vi "Program.vi"() -> ()   [LabVIEW 2026]
uses:
  <instrlib>/MicroPulse/Public/Data/Datatypes/MP - pulse damping.ctl
  <instrlib>/MicroPulse/Public/Data/Datatypes/MP - frequency filter.ctl
  <instrlib>/MicroPulse/Public/Data/Datatypes/MP - sample frequency.ctl
  <instrlib>/MicroPulse/Public/Data/Datatypes/TCP config.ctl
  <instrlib>/MicroPulse/Public/Data/Datatypes/MP - test parameters.ctl
  <instrlib>/MicroPulse/Public/Data/Datatypes/MP - transmit parameters.ctl
  <instrlib>/MicroPulse/Public/Data/Datatypes/MP - pulser voltage.ctl
  <instrlib>/MicroPulse/Public/Data/Datatypes/MP - receive parameters.ctl
  <instrlib>/MicroPulse/Public/Data/Datatypes/MP - display gate.ctl
  <instrlib>/MicroPulse/Public/Data/Datatypes/MP - waveform type.ctl
  <instrlib>/MicroPulse/Public/Data/Datatypes/MP - analogue filter.ctl
  <instrlib>/MicroPulse/Public/Data/Datatypes/MP - digital filtering.ctl
  <instrlib>/MicroPulse/Public/Data/Datatypes/MP - high pass filter.ctl
  <instrlib>/MicroPulse/Public/Data/Datatypes/MP - low pass filter.ctl
  <instrlib>/MicroPulse/Public/Data/Datatypes/MP - multi-gate inspection.ctl
  <instrlib>/MicroPulse/Public/Data/Datatypes/MP - multigate inspection gate parameters.ctl
  <instrlib>/MicroPulse/Public/Data/Datatypes/MP - hysteresis level.ctl
  <instrlib>/MicroPulse/Public/Data/Datatypes/MP - multigate mode.ctl
  <instrlib>/MicroPulse/Public/Data/Datatypes/MP - data formatting.ctl
  <instrlib>/MicroPulse/Public/Data/Datatypes/MP - amplitude reporting mode.ctl
  <instrlib>/MicroPulse/Public/Data/Datatypes/MP - averaging.ctl
  <vilib>/ErrorRing/Error Ring.xnode
  <instrlib>/MicroPulse/MicroPulse_Driver.lvlib
panel:
  in  "Main Tab Control":T1(tab)
  in  "Calculate Scan":bool
  in  "Scan Information":T2 {"Date" format="%<%x>T"}
  in  "Scan Settings":T3={"Selected Beam X"=0.0, "Enabled Channels"=1.0, "Scan Data Rate"=0.0, "Scan Resolution"=0.0, "Scan Speed (deg/s)"=0.0, "Scan RPM"=0.0, "Pulses Per Rev"=0.0} {"Enabled Channels" min=1.0 max=7.0 step=1.0 format="%#.0f"}
  in  "Transducer Information":string[][](table)
  in  "Gain Slider":dbl(slide) caption="Gain (dB)" min=0.0 max=50.0 step=0.25 scale=0.0..50.0
  in  "Channel Setup Tab Control":T4(tab)
  in  "Pulse Width Damping Channel 1":T7
  in  "Interface Channel 1":T8
  out "Flaw Indicators Channel 1":T9
  in  "Flaw Gate Channel 1":T8 caption="Flaw Gate (mm Ti)"
  in  "Backwall Gate Channel 1":T8 caption="Backwall Gate (mm)"
  in  "A-Scan Window Channel 1":cluster{"Start":dbl, "Range":dbl} caption="A-Scan Window (mm)"
  in  "Pulse Width Damping Channel 2":T7
  in  "Interface Channel 2":T8
  out "Flaw Indicators Channel 2":T9
  in  "Flaw Gate Channel 2":T8 caption="Flaw Gate (mm Ti)"
  in  "Backwall Gate Channel 2":T8 caption="Backwall Gate (mm)"
  in  "A-Scan Window Channel 2":cluster{"Start":dbl, "Range":dbl} caption="A-Scan Window (mm)"
  in  "Pulse Width Damping Channel 3":T7
  in  "Interface Channel 3":T8
  out "Flaw Indicators Channel 3":T9
  in  "Flaw Gate Channel 3":T8 caption="Flaw Gate (mm Ti)"
  in  "Backwall Gate Channel 3":T8 caption="Backwall Gate (mm)"
  in  "A-Scan Window Channel 3":cluster{"Start":dbl, "Range":dbl} caption="A-Scan Window (mm)"
  in  "A-Scan Window Channel 4":cluster{"Start":dbl, "Range":dbl} caption="A-Scan Window (mm)"
  in  "Backwall Gate Channel 4":T8 caption="Backwall Gate (mm)"
  in  "Flaw Gate Channel 4":T8 caption="Flaw Gate (mm Ti)"
  out "Flaw Indicators Channel 4":T9
  in  "Interface Channel 4":T8
  in  "Pulse Width Damping Channel 4":T7
  in  "Pulse Width Damping Channel 5":T7
  in  "Interface Channel 5":T8
  out "Flaw Indicators Channel 5":T9
  in  "Flaw Gate Channel 5":T8 caption="Flaw Gate (mm Ti)"
  in  "Backwall Gate Channel 5":T8 caption="Backwall Gate (mm)"
  in  "A-Scan Window Channel 5":cluster{"Start":dbl, "Range":dbl} caption="A-Scan Window (mm)"
  in  "Pulse Width Damping Channel 6":T7
  in  "Interface Channel 6":T8
  out "Flaw Indicators Channel 6":T9
  in  "Flaw Gate Channel 6":T8 caption="Flaw Gate (mm Ti)"
  in  "Backwall Gate Channel 6":T8 caption="Backwall Gate (mm)"
  in  "A-Scan Window Channel 6":cluster{"Start":dbl, "Range":dbl} caption="A-Scan Window (mm)"
  in  "Pulse Width Damping Channel 7":T7
  in  "Interface Channel 7":T8
  out "Flaw Indicators Channel 7":T9
  in  "Flaw Gate Channel 7":T8 caption="Flaw Gate (mm Ti)"
  in  "Backwall Gate Channel 7":T8 caption="Backwall Gate (mm)"
  in  "A-Scan Window Channel 7":cluster{"Start":dbl, "Range":dbl} caption="A-Scan Window (mm)"
  out "Channel Setup Graph":cluster{"timebase":dbl[], "data":u16[]}[](graph)
  in  "Channel Select":T10(ring)
  in  "Channel Variables Tab Control":T4(tab)
  in  "RX Channel 1":T11 {"Delay" format="%#_g us"; "Display Gate"."Length" min=0.0 max=64000.0 step=1.0 format="%#_g us"; "Display Gate"."Start" min=0.0 max=64000.0 step=1.0 format="%#_g us"; "Analogue Filtering"."Smoothing" min=1 max=11 step=1; "Gain" min=-6.0 max=70.0 step=0.25 format="%.2fdB"}
  in  "Test Channel 1":T18={"Test No."=1, "Tx Channel"=1, "Rx Channel"=1} {"Rx Channel" min=1 max=1024; "Tx Channel" min=1 max=1024}
  in  "TX Channel 1":T19 {"Pulse Shape"."Width" min=16 max=1010 step=50 format="%.0fns"}
  in  "Data Format Channel 1":T21={"Amplitude Mode"=enum."Peaks + Ascan for Multigate", "Averaging"=enum."None", "Coupling Level"=0} {"Coupling Level" max=4095 step=1}
  in  "Gates Channel 1":T24={"Gate 1"={"Start (us)"=0.0, "Length (us)"=0.0, "Threshold"=10, "Enabled?"=FALSE, "Max # Peaks"=0, "Hysteresis"=enum."None", "Mode"=enum."1st Peak in Gate", "Inverted?"=FALSE, "Colour "=0}, "Gate 2"={"Start (us)"=0.0, "Length (us)"=0.0, "Threshold"=10, "Enabled?"=FALSE, "Max # Peaks"=0, "Hysteresis"=enum."None", "Mode"=enum."1st Peak in Gate", "Inverted?"=FALSE, "Colour "=0}, "Gate 3"={"Start (us)"=0.0, "Length (us)"=0.0, "Threshold"=10, "Enabled?"=FALSE, "Max # Peaks"=0, "Hysteresis"=enum."None", "Mode"=enum."1st Peak in Gate", "Inverted?"=FALSE, "Colour "=0}, "Gate 4"={"Start (us)"=0.0, "Length (us)"=0.0, "Threshold"=10, "Enabled?"=FALSE, "Max # Peaks"=0, "Hysteresis"=enum."None", "Mode"=enum."1st Peak in Gate", "Inverted?"=FALSE, "Colour "=0}} {"Gate 4"."Max # Peaks" max=64000 step=100; "Gate 4"."Threshold" min=10 max=4095 step=10; "Gate 4"."Length (us)" min=0.0 max=96000.0 step=100.0; "Gate 4"."Start (us)" min=0.0 max=64000.0 step=100.0; "Gate 3"."Max # Peaks" max=64000 step=100; "Gate 3"."Threshold" min=10 max=4095 step=10; "Gate 3"."Length (us)" min=0.0 max=96000.0 step=100.0; "Gate 3"."Start (us)" min=0.0 max=64000.0 step=100.0; "Gate 2"."Max # Peaks" max=64000 step=100; "Gate 2"."Threshold" min=10 max=4095 step=10; "Gate 2"."Length (us)" min=0.0 max=96000.0 step=100.0; "Gate 2"."Start (us)" min=0.0 max=64000.0 step=100.0; "Gate 1"."Max # Peaks" max=64000 step=100; "Gate 1"."Threshold" min=10 max=4095 step=10; "Gate 1"."Length (us)" min=0.0 max=96000.0 step=100.0; "Gate 1"."Start (us)" min=0.0 max=64000.0 step=100.0}
  in  "Gates Channel 2":T24={"Gate 1"={"Start (us)"=0.0, "Length (us)"=0.0, "Threshold"=10, "Enabled?"=FALSE, "Max # Peaks"=0, "Hysteresis"=enum."None", "Mode"=enum."1st Peak in Gate", "Inverted?"=FALSE, "Colour "=0}, "Gate 2"={"Start (us)"=0.0, "Length (us)"=0.0, "Threshold"=10, "Enabled?"=FALSE, "Max # Peaks"=0, "Hysteresis"=enum."None", "Mode"=enum."1st Peak in Gate", "Inverted?"=FALSE, "Colour "=0}, "Gate 3"={"Start (us)"=0.0, "Length (us)"=0.0, "Threshold"=10, "Enabled?"=FALSE, "Max # Peaks"=0, "Hysteresis"=enum."None", "Mode"=enum."1st Peak in Gate", "Inverted?"=FALSE, "Colour "=0}, "Gate 4"={"Start (us)"=0.0, "Length (us)"=0.0, "Threshold"=10, "Enabled?"=FALSE, "Max # Peaks"=0, "Hysteresis"=enum."None", "Mode"=enum."1st Peak in Gate", "Inverted?"=FALSE, "Colour "=0}} {"Gate 4"."Max # Peaks" max=64000 step=100; "Gate 4"."Threshold" min=10 max=4095 step=10; "Gate 4"."Length (us)" min=0.0 max=96000.0 step=100.0; "Gate 4"."Start (us)" min=0.0 max=64000.0 step=100.0; "Gate 3"."Max # Peaks" max=64000 step=100; "Gate 3"."Threshold" min=10 max=4095 step=10; "Gate 3"."Length (us)" min=0.0 max=96000.0 step=100.0; "Gate 3"."Start (us)" min=0.0 max=64000.0 step=100.0; "Gate 2"."Max # Peaks" max=64000 step=100; "Gate 2"."Threshold" min=10 max=4095 step=10; "Gate 2"."Length (us)" min=0.0 max=96000.0 step=100.0; "Gate 2"."Start (us)" min=0.0 max=64000.0 step=100.0; "Gate 1"."Max # Peaks" max=64000 step=100; "Gate 1"."Threshold" min=10 max=4095 step=10; "Gate 1"."Length (us)" min=0.0 max=96000.0 step=100.0; "Gate 1"."Start (us)" min=0.0 max=64000.0 step=100.0}
  in  "Data Format Channel 2":T21={"Amplitude Mode"=enum."Peaks + Ascan for Multigate", "Averaging"=enum."None", "Coupling Level"=0} {"Coupling Level" max=4095 step=1}
  in  "TX Channel 2":T19 {"Pulse Shape"."Width" min=16 max=1010 step=50 format="%.0fns"}
  in  "Test Channel 2":T18={"Test No."=2, "Tx Channel"=2, "Rx Channel"=2} {"Rx Channel" min=1 max=1024; "Tx Channel" min=1 max=1024}
  in  "RX Channel 2":T11 {"Delay" format="%#_g us"; "Display Gate"."Length" min=0.0 max=64000.0 step=1.0 format="%#_g us"; "Display Gate"."Start" min=0.0 max=64000.0 step=1.0 format="%#_g us"; "Analogue Filtering"."Smoothing" min=1 max=11 step=1; "Gain" min=-6.0 max=70.0 step=0.25 format="%.2fdB"}
  in  "Gates Channel 3":T24={"Gate 1"={"Start (us)"=0.0, "Length (us)"=0.0, "Threshold"=10, "Enabled?"=FALSE, "Max # Peaks"=0, "Hysteresis"=enum."None", "Mode"=enum."1st Peak in Gate", "Inverted?"=FALSE, "Colour "=0}, "Gate 2"={"Start (us)"=0.0, "Length (us)"=0.0, "Threshold"=10, "Enabled?"=FALSE, "Max # Peaks"=0, "Hysteresis"=enum."None", "Mode"=enum."1st Peak in Gate", "Inverted?"=FALSE, "Colour "=0}, "Gate 3"={"Start (us)"=0.0, "Length (us)"=0.0, "Threshold"=10, "Enabled?"=FALSE, "Max # Peaks"=0, "Hysteresis"=enum."None", "Mode"=enum."1st Peak in Gate", "Inverted?"=FALSE, "Colour "=0}, "Gate 4"={"Start (us)"=0.0, "Length (us)"=0.0, "Threshold"=10, "Enabled?"=FALSE, "Max # Peaks"=0, "Hysteresis"=enum."None", "Mode"=enum."1st Peak in Gate", "Inverted?"=FALSE, "Colour "=0}} {"Gate 4"."Max # Peaks" max=64000 step=100; "Gate 4"."Threshold" min=10 max=4095 step=10; "Gate 4"."Length (us)" min=0.0 max=96000.0 step=100.0; "Gate 4"."Start (us)" min=0.0 max=64000.0 step=100.0; "Gate 3"."Max # Peaks" max=64000 step=100; "Gate 3"."Threshold" min=10 max=4095 step=10; "Gate 3"."Length (us)" min=0.0 max=96000.0 step=100.0; "Gate 3"."Start (us)" min=0.0 max=64000.0 step=100.0; "Gate 2"."Max # Peaks" max=64000 step=100; "Gate 2"."Threshold" min=10 max=4095 step=10; "Gate 2"."Length (us)" min=0.0 max=96000.0 step=100.0; "Gate 2"."Start (us)" min=0.0 max=64000.0 step=100.0; "Gate 1"."Max # Peaks" max=64000 step=100; "Gate 1"."Threshold" min=10 max=4095 step=10; "Gate 1"."Length (us)" min=0.0 max=96000.0 step=100.0; "Gate 1"."Start (us)" min=0.0 max=64000.0 step=100.0}
  in  "Data Format Channel 3":T21={"Amplitude Mode"=enum."Peaks + Ascan for Multigate", "Averaging"=enum."None", "Coupling Level"=0} {"Coupling Level" max=4095 step=1}
  in  "TX Channel 3":T19 {"Pulse Shape"."Width" min=16 max=1010 step=50 format="%.0fns"}
  in  "Test Channel 3":T18={"Test No."=3, "Tx Channel"=3, "Rx Channel"=3} {"Rx Channel" min=1 max=1024; "Tx Channel" min=1 max=1024}
  in  "RX Channel 3":T11 {"Delay" format="%#_g us"; "Display Gate"."Length" min=0.0 max=64000.0 step=1.0 format="%#_g us"; "Display Gate"."Start" min=0.0 max=64000.0 step=1.0 format="%#_g us"; "Analogue Filtering"."Smoothing" min=1 max=11 step=1; "Gain" min=-6.0 max=70.0 step=0.25 format="%.2fdB"}
  in  "RX Channel 4":T11 {"Delay" format="%#_g us"; "Display Gate"."Length" min=0.0 max=64000.0 step=1.0 format="%#_g us"; "Display Gate"."Start" min=0.0 max=64000.0 step=1.0 format="%#_g us"; "Analogue Filtering"."Smoothing" min=1 max=11 step=1; "Gain" min=-6.0 max=70.0 step=0.25 format="%.2fdB"}
  in  "Test Channel 4":T18={"Test No."=4, "Tx Channel"=4, "Rx Channel"=4} {"Rx Channel" min=1 max=1024; "Tx Channel" min=1 max=1024}
  in  "TX Channel 4":T19 {"Pulse Shape"."Width" min=16 max=1010 step=50 format="%.0fns"}
  in  "Data Format Channel 4":T21={"Amplitude Mode"=enum."Peaks + Ascan for Multigate", "Averaging"=enum."None", "Coupling Level"=0} {"Coupling Level" max=4095 step=1}
  in  "Gates Channel 4":T24={"Gate 1"={"Start (us)"=0.0, "Length (us)"=0.0, "Threshold"=10, "Enabled?"=FALSE, "Max # Peaks"=0, "Hysteresis"=enum."None", "Mode"=enum."1st Peak in Gate", "Inverted?"=FALSE, "Colour "=0}, "Gate 2"={"Start (us)"=0.0, "Length (us)"=0.0, "Threshold"=10, "Enabled?"=FALSE, "Max # Peaks"=0, "Hysteresis"=enum."None", "Mode"=enum."1st Peak in Gate", "Inverted?"=FALSE, "Colour "=0}, "Gate 3"={"Start (us)"=0.0, "Length (us)"=0.0, "Threshold"=10, "Enabled?"=FALSE, "Max # Peaks"=0, "Hysteresis"=enum."None", "Mode"=enum."1st Peak in Gate", "Inverted?"=FALSE, "Colour "=0}, "Gate 4"={"Start (us)"=0.0, "Length (us)"=0.0, "Threshold"=10, "Enabled?"=FALSE, "Max # Peaks"=0, "Hysteresis"=enum."None", "Mode"=enum."1st Peak in Gate", "Inverted?"=FALSE, "Colour "=0}} {"Gate 4"."Max # Peaks" max=64000 step=100; "Gate 4"."Threshold" min=10 max=4095 step=10; "Gate 4"."Length (us)" min=0.0 max=96000.0 step=100.0; "Gate 4"."Start (us)" min=0.0 max=64000.0 step=100.0; "Gate 3"."Max # Peaks" max=64000 step=100; "Gate 3"."Threshold" min=10 max=4095 step=10; "Gate 3"."Length (us)" min=0.0 max=96000.0 step=100.0; "Gate 3"."Start (us)" min=0.0 max=64000.0 step=100.0; "Gate 2"."Max # Peaks" max=64000 step=100; "Gate 2"."Threshold" min=10 max=4095 step=10; "Gate 2"."Length (us)" min=0.0 max=96000.0 step=100.0; "Gate 2"."Start (us)" min=0.0 max=64000.0 step=100.0; "Gate 1"."Max # Peaks" max=64000 step=100; "Gate 1"."Threshold" min=10 max=4095 step=10; "Gate 1"."Length (us)" min=0.0 max=96000.0 step=100.0; "Gate 1"."Start (us)" min=0.0 max=64000.0 step=100.0}
  in  "RX Channel 5":T11 {"Delay" format="%#_g us"; "Display Gate"."Length" min=0.0 max=64000.0 step=1.0 format="%#_g us"; "Display Gate"."Start" min=0.0 max=64000.0 step=1.0 format="%#_g us"; "Analogue Filtering"."Smoothing" min=1 max=11 step=1; "Gain" min=-6.0 max=70.0 step=0.25 format="%.2fdB"}
  in  "Test Channel 5":T18={"Test No."=5, "Tx Channel"=5, "Rx Channel"=5} {"Rx Channel" min=1 max=1024; "Tx Channel" min=1 max=1024}
  in  "TX Channel 5":T19 {"Pulse Shape"."Width" min=16 max=1010 step=50 format="%.0fns"}
  in  "Data Format Channel 5":T21={"Amplitude Mode"=enum."Peaks + Ascan for Multigate", "Averaging"=enum."None", "Coupling Level"=0} {"Coupling Level" max=4095 step=1}
  in  "Gates Channel 5":T24={"Gate 1"={"Start (us)"=0.0, "Length (us)"=0.0, "Threshold"=10, "Enabled?"=FALSE, "Max # Peaks"=0, "Hysteresis"=enum."None", "Mode"=enum."1st Peak in Gate", "Inverted?"=FALSE, "Colour "=0}, "Gate 2"={"Start (us)"=0.0, "Length (us)"=0.0, "Threshold"=10, "Enabled?"=FALSE, "Max # Peaks"=0, "Hysteresis"=enum."None", "Mode"=enum."1st Peak in Gate", "Inverted?"=FALSE, "Colour "=0}, "Gate 3"={"Start (us)"=0.0, "Length (us)"=0.0, "Threshold"=10, "Enabled?"=FALSE, "Max # Peaks"=0, "Hysteresis"=enum."None", "Mode"=enum."1st Peak in Gate", "Inverted?"=FALSE, "Colour "=0}, "Gate 4"={"Start (us)"=0.0, "Length (us)"=0.0, "Threshold"=10, "Enabled?"=FALSE, "Max # Peaks"=0, "Hysteresis"=enum."None", "Mode"=enum."1st Peak in Gate", "Inverted?"=FALSE, "Colour "=0}} {"Gate 4"."Max # Peaks" max=64000 step=100; "Gate 4"."Threshold" min=10 max=4095 step=10; "Gate 4"."Length (us)" min=0.0 max=96000.0 step=100.0; "Gate 4"."Start (us)" min=0.0 max=64000.0 step=100.0; "Gate 3"."Max # Peaks" max=64000 step=100; "Gate 3"."Threshold" min=10 max=4095 step=10; "Gate 3"."Length (us)" min=0.0 max=96000.0 step=100.0; "Gate 3"."Start (us)" min=0.0 max=64000.0 step=100.0; "Gate 2"."Max # Peaks" max=64000 step=100; "Gate 2"."Threshold" min=10 max=4095 step=10; "Gate 2"."Length (us)" min=0.0 max=96000.0 step=100.0; "Gate 2"."Start (us)" min=0.0 max=64000.0 step=100.0; "Gate 1"."Max # Peaks" max=64000 step=100; "Gate 1"."Threshold" min=10 max=4095 step=10; "Gate 1"."Length (us)" min=0.0 max=96000.0 step=100.0; "Gate 1"."Start (us)" min=0.0 max=64000.0 step=100.0}
  in  "RX Channel 6":T11 {"Delay" format="%#_g us"; "Display Gate"."Length" min=0.0 max=64000.0 step=1.0 format="%#_g us"; "Display Gate"."Start" min=0.0 max=64000.0 step=1.0 format="%#_g us"; "Analogue Filtering"."Smoothing" min=1 max=11 step=1; "Gain" min=-6.0 max=70.0 step=0.25 format="%.2fdB"}
  in  "Test Channel 6":T18={"Test No."=6, "Tx Channel"=6, "Rx Channel"=6} {"Rx Channel" min=1 max=1024; "Tx Channel" min=1 max=1024}
  in  "TX Channel 6":T19 {"Pulse Shape"."Width" min=16 max=1010 step=50 format="%.0fns"}
  in  "Data Format Channel 6":T21={"Amplitude Mode"=enum."Peaks + Ascan for Multigate", "Averaging"=enum."None", "Coupling Level"=0} {"Coupling Level" max=4095 step=1}
  in  "Gates Channel 6":T24={"Gate 1"={"Start (us)"=0.0, "Length (us)"=0.0, "Threshold"=10, "Enabled?"=FALSE, "Max # Peaks"=0, "Hysteresis"=enum."None", "Mode"=enum."1st Peak in Gate", "Inverted?"=FALSE, "Colour "=0}, "Gate 2"={"Start (us)"=0.0, "Length (us)"=0.0, "Threshold"=10, "Enabled?"=FALSE, "Max # Peaks"=0, "Hysteresis"=enum."None", "Mode"=enum."1st Peak in Gate", "Inverted?"=FALSE, "Colour "=0}, "Gate 3"={"Start (us)"=0.0, "Length (us)"=0.0, "Threshold"=10, "Enabled?"=FALSE, "Max # Peaks"=0, "Hysteresis"=enum."None", "Mode"=enum."1st Peak in Gate", "Inverted?"=FALSE, "Colour "=0}, "Gate 4"={"Start (us)"=0.0, "Length (us)"=0.0, "Threshold"=10, "Enabled?"=FALSE, "Max # Peaks"=0, "Hysteresis"=enum."None", "Mode"=enum."1st Peak in Gate", "Inverted?"=FALSE, "Colour "=0}} {"Gate 4"."Max # Peaks" max=64000 step=100; "Gate 4"."Threshold" min=10 max=4095 step=10; "Gate 4"."Length (us)" min=0.0 max=96000.0 step=100.0; "Gate 4"."Start (us)" min=0.0 max=64000.0 step=100.0; "Gate 3"."Max # Peaks" max=64000 step=100; "Gate 3"."Threshold" min=10 max=4095 step=10; "Gate 3"."Length (us)" min=0.0 max=96000.0 step=100.0; "Gate 3"."Start (us)" min=0.0 max=64000.0 step=100.0; "Gate 2"."Max # Peaks" max=64000 step=100; "Gate 2"."Threshold" min=10 max=4095 step=10; "Gate 2"."Length (us)" min=0.0 max=96000.0 step=100.0; "Gate 2"."Start (us)" min=0.0 max=64000.0 step=100.0; "Gate 1"."Max # Peaks" max=64000 step=100; "Gate 1"."Threshold" min=10 max=4095 step=10; "Gate 1"."Length (us)" min=0.0 max=96000.0 step=100.0; "Gate 1"."Start (us)" min=0.0 max=64000.0 step=100.0}
  in  "RX Channel 7":T11 {"Delay" format="%#_g us"; "Display Gate"."Length" min=0.0 max=64000.0 step=1.0 format="%#_g us"; "Display Gate"."Start" min=0.0 max=64000.0 step=1.0 format="%#_g us"; "Analogue Filtering"."Smoothing" min=1 max=11 step=1; "Gain" min=-6.0 max=70.0 step=0.25 format="%.2fdB"}
  in  "Test Channel 7":T18={"Test No."=7, "Tx Channel"=7, "Rx Channel"=7} {"Rx Channel" min=1 max=1024; "Tx Channel" min=1 max=1024}
  in  "TX Channel 7":T19 {"Pulse Shape"."Width" min=16 max=1010 step=50 format="%.0fns"}
  in  "Data Format Channel 7":T21={"Amplitude Mode"=enum."Peaks + Ascan for Multigate", "Averaging"=enum."None", "Coupling Level"=0} {"Coupling Level" max=4095 step=1}
  in  "Gates Channel 7":T24={"Gate 1"={"Start (us)"=0.0, "Length (us)"=0.0, "Threshold"=10, "Enabled?"=FALSE, "Max # Peaks"=0, "Hysteresis"=enum."None", "Mode"=enum."1st Peak in Gate", "Inverted?"=FALSE, "Colour "=0}, "Gate 2"={"Start (us)"=0.0, "Length (us)"=0.0, "Threshold"=10, "Enabled?"=FALSE, "Max # Peaks"=0, "Hysteresis"=enum."None", "Mode"=enum."1st Peak in Gate", "Inverted?"=FALSE, "Colour "=0}, "Gate 3"={"Start (us)"=0.0, "Length (us)"=0.0, "Threshold"=10, "Enabled?"=FALSE, "Max # Peaks"=0, "Hysteresis"=enum."None", "Mode"=enum."1st Peak in Gate", "Inverted?"=FALSE, "Colour "=0}, "Gate 4"={"Start (us)"=0.0, "Length (us)"=0.0, "Threshold"=10, "Enabled?"=FALSE, "Max # Peaks"=0, "Hysteresis"=enum."None", "Mode"=enum."1st Peak in Gate", "Inverted?"=FALSE, "Colour "=0}} {"Gate 4"."Max # Peaks" max=64000 step=100; "Gate 4"."Threshold" min=10 max=4095 step=10; "Gate 4"."Length (us)" min=0.0 max=96000.0 step=100.0; "Gate 4"."Start (us)" min=0.0 max=64000.0 step=100.0; "Gate 3"."Max # Peaks" max=64000 step=100; "Gate 3"."Threshold" min=10 max=4095 step=10; "Gate 3"."Length (us)" min=0.0 max=96000.0 step=100.0; "Gate 3"."Start (us)" min=0.0 max=64000.0 step=100.0; "Gate 2"."Max # Peaks" max=64000 step=100; "Gate 2"."Threshold" min=10 max=4095 step=10; "Gate 2"."Length (us)" min=0.0 max=96000.0 step=100.0; "Gate 2"."Start (us)" min=0.0 max=64000.0 step=100.0; "Gate 1"."Max # Peaks" max=64000 step=100; "Gate 1"."Threshold" min=10 max=4095 step=10; "Gate 1"."Length (us)" min=0.0 max=96000.0 step=100.0; "Gate 1"."Start (us)" min=0.0 max=64000.0 step=100.0}
  in  "MicroPulse Initialise":T30={"Hard Reset?"=FALSE, "Sample Frequency"=enum."Use Default", "TCP config"={"Connection ID"=refnum, "IP address"="10.1.1.2", "host port"=1067, "OC timeout"=-1, "Read timeout"=0, "Write timeout"=0}, "PRF (Hz)"=0.0} {"TCP config"."Write timeout" format="%dms"; "TCP config"."Read timeout" format="%dms"; "TCP config"."OC timeout" format="%dms"}
  out "Key Held":bool
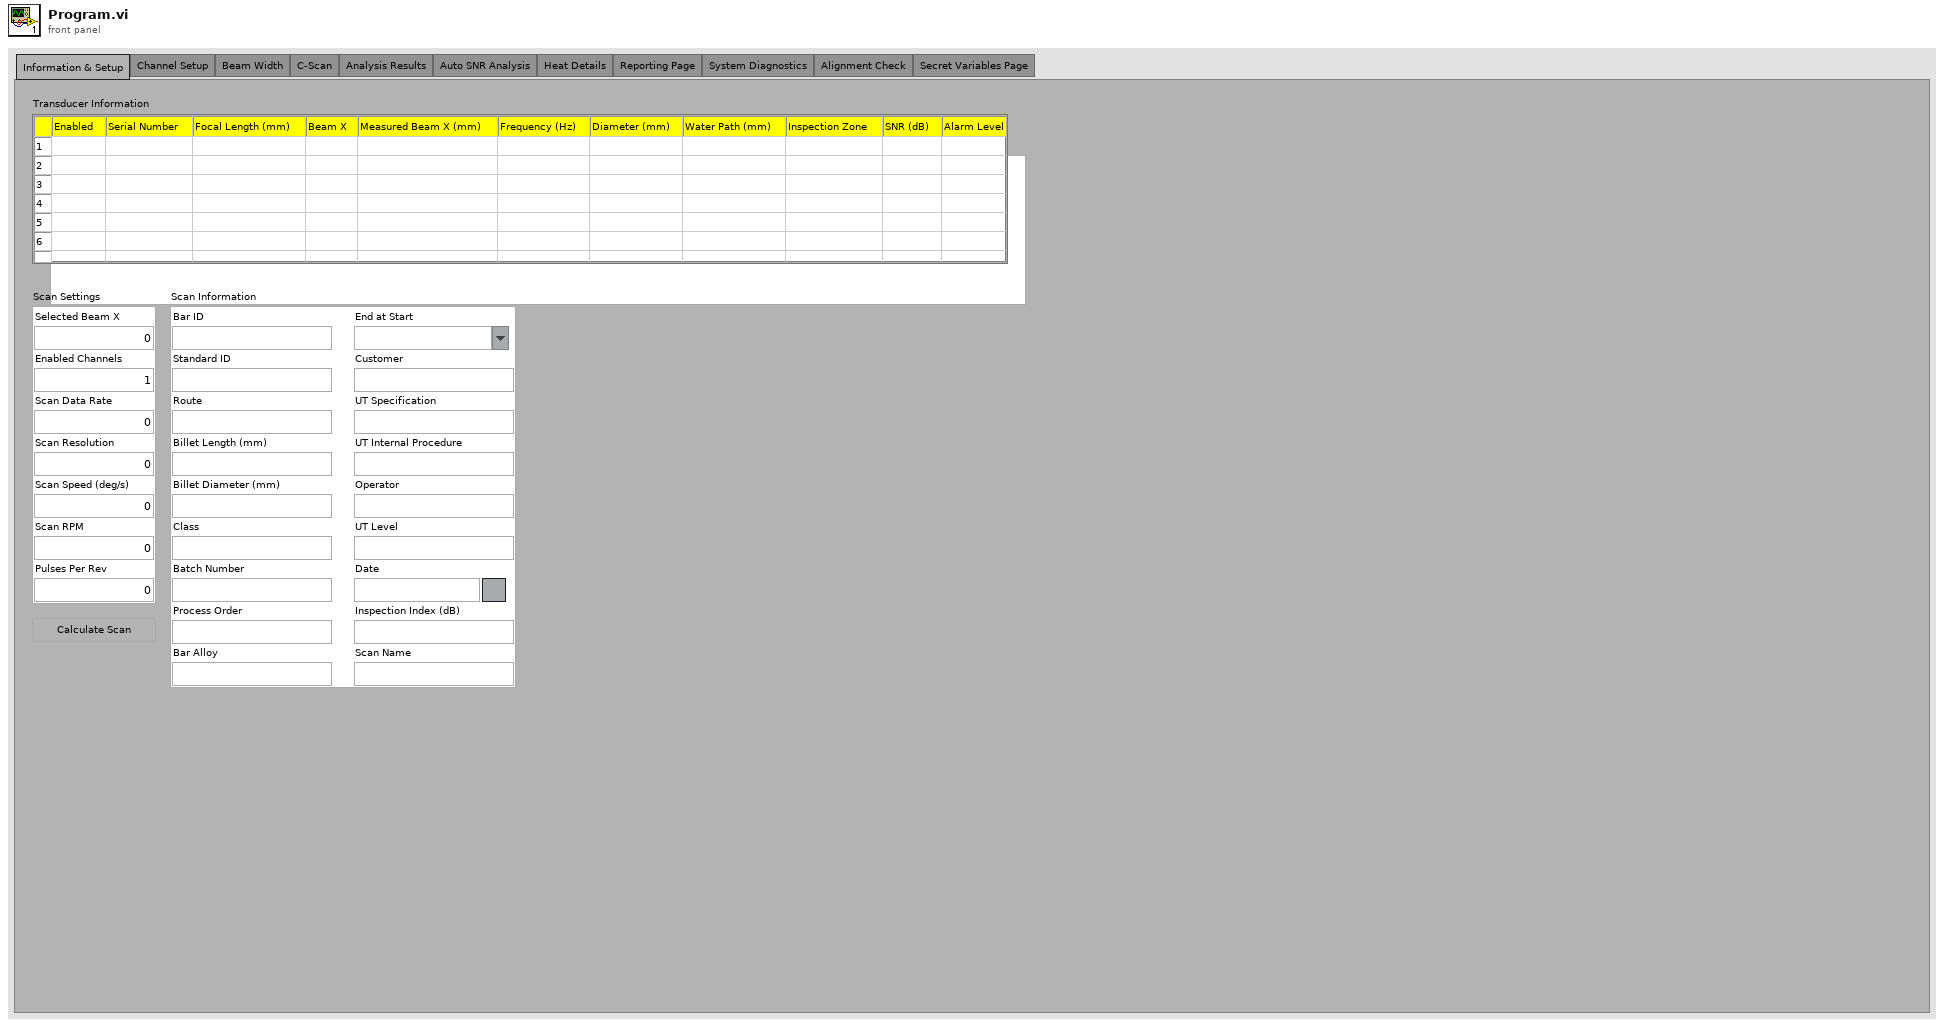
[diagram p1: front panel]
types:
  T1 = enum32{"Information & Setup", "Channel Setup", "Beam Width", "C-Scan", "Analysis Results", "Auto SNR Analysis", "Heat Details", "Reporting Page", "System Diagnostics", "Alignment Check", "Secret Variables Page"}
  T2 = cluster{"Bar ID":string, "Standard ID":string, "Route":string, "Billet Length (mm)":dbl, "Billet Diameter (mm)":dbl, "Class":string, "Batch Number":string, "Process Order":string, "Bar Alloy":string, "Scan Name":string, "Inspection Index (dB)":enum16{""}, "Date":timestamp, "UT Level":string, "Operator":string, "UT Internal Procedure":string, "UT Specification":string, "Customer":string, "End at Start":string}
  T3 = cluster{"Selected Beam X":dbl, "Enabled Channels":dbl, "Scan Data Rate":dbl, "Scan Resolution":dbl, "Scan Speed (deg/s)":dbl, "Scan RPM":dbl, "Pulses Per Rev":dbl}
  T4 = enum32{"Channel 1", "Channel 2", "Channel 3", "Channel 4", "Channel 5", "Channel 6", "Channel 7"}
  T5 = typedef "MicroPulse_Driver.lvlib/MP - pulse damping.ctl" = enum16{"660W", "458W", "220W", "149W", "102W", "82W", "63W", "51W"}
  T6 = typedef "MicroPulse_Driver.lvlib/MP - frequency filter.ctl" = enum16{"No change", "1MHz Bandpass", "2MHz Bandpass", "4MHz Bandpass", "5MHz Bandpass", "10MHz Bandpass", "2.5-18MHz Broadband", "0.75-12MHz  Broadband", "0.5MHz Bandpass", "5MHz 2nd Order TOFD", "10MHz 2nd Order TOFD", "3.0-25MHz Broadband", "3.0-30MHz Broadband"}
  T7 = cluster{"Pulse Width":dbl, "Damping Channel 1":T5, "Rectification":enum16{"Rectified Signal", "RF Signal", "+Half Wave", "-Half Wave"}, "Filter":T6}
  T8 = cluster{"Start":dbl, "Length":dbl, "Threshold":dbl}
  T9 = cluster{"Water Path":dbl, "Gate AMP":dbl, "Gate TOF":dbl}
  T10 = enum16{"Channel 1", "Channel 2", "Channel 3", "Channel 4", "Channel 5", "Channel 6", "Channel 7"}
  T11 = typedef "MicroPulse_Driver.lvlib/MP - receive parameters.ctl" = cluster{"Display Gate":T12, "Delay":dbl, "Waveform Type":T13, "Gain":dbl, "Analogue Filtering":T14, "Digital Filtering":T15}
  T12 = typedef "MicroPulse_Driver.lvlib/MP - display gate.ctl" = cluster{"Start":dbl, "Length":dbl}
  T13 = typedef "MicroPulse_Driver.lvlib/MP - waveform type.ctl" = enum16{"Rectified Signal", "RF Signal", "+Half Wave", "-Half Wave"}
  T14 = typedef "MicroPulse_Driver.lvlib/MP - analogue filter.ctl" = cluster{"Bandpass":T6, "Smoothing":u16}
  T15 = typedef "MicroPulse_Driver.lvlib/MP - digital filtering.ctl" = cluster{"High Pass Filter":T16, "Low Pass Filter":T17}
  T16 = typedef "MicroPulse_Driver.lvlib/MP - high pass filter.ctl" = enum16{"None", "0.7MHz", "1.5MHz", "4.0MHz", "7.5MHz", "10.0MHz", "User Defined"}
  T17 = typedef "MicroPulse_Driver.lvlib/MP - low pass filter.ctl" = enum16{"None", "1.8MHz", "3.0MHz", "6.0MHz", "8.0MHz", "12.0MHz", "User Defined"}
  T18 = typedef "MicroPulse_Driver.lvlib/MP - test parameters.ctl" = cluster{"Test No.":u32, "Tx Channel":u32, "Rx Channel":u32}
  T19 = typedef "MicroPulse_Driver.lvlib/MP - transmit parameters.ctl" = cluster{"Pulse Voltage":T20, "Pulse Shape":cluster{"Damping":T5, "Width":u32}}
  T20 = typedef "MicroPulse_Driver.lvlib/MP - pulser voltage.ctl" = enum16{"50V", "100V", "150V", "200V", "250V", "300V"}
  T21 = typedef "MicroPulse_Driver.lvlib/MP - data formatting.ctl" = cluster{"Amplitude Mode":T22, "Averaging":T23, "Coupling Level":u32}
  T22 = typedef "MicroPulse_Driver.lvlib/MP - amplitude reporting mode.ctl" = enum16{"1st Peak in gate", "Maximum Peak in gate", "All Peaks", "Ascan Data", "1st Threshold Crossing Peak", "Ascan + Peaks", "All Peaks for Multigate", "Peaks + Ascan for Multigate", "Peaks + P_Ascan for Multigate", "Full Matrix Capture"}
  T23 = typedef "MicroPulse_Driver.lvlib/MP - averaging.ctl" = enum16{"None", "2", "4", "8", "16", "32", "64", "128", "256"}
  T24 = typedef "MicroPulse_Driver.lvlib/MP - multi-gate inspection.ctl" = cluster{"Gate 1":T25, "Gate 2":T25, "Gate 3":T25, "Gate 4":T25}
  T25 = typedef "MicroPulse_Driver.lvlib/MP - multigate inspection gate parameters.ctl" = cluster{"Start (us)":dbl, "Length (us)":dbl, "Threshold":u16, "Enabled?":bool, "Max # Peaks":u16, "Hysteresis":T26, "Mode":T27, "Inverted?":bool, "Colour ":u32}
  T26 = typedef "MicroPulse_Driver.lvlib/MP - hysteresis level.ctl" = enum16{"None", "3dB", "6dB", "9dB", "12dB"}
  T27 = typedef "MicroPulse_Driver.lvlib/MP - multigate mode.ctl" = enum16{"1st Peak in Gate", "Largest Peak In Gate", "All Peaks In Gate", "1st Threshold Crossing"}
  T28 = typedef "MicroPulse_Driver.lvlib/MP - sample frequency.ctl" = enum16{"Use Default", "200MHz (LT2 only)", "100MHz", "50MHz", "25MHz", "10MHz"}
  T29 = typedef "MicroPulse_Driver.lvlib/TCP config.ctl" = cluster{"Connection ID":refnum<k5>, "IP address":string, "host port":u16, "OC timeout":i32, "Read timeout":i32, "Write timeout":i32}
  T30 = cluster{"Hard Reset?":bool, "Sample Frequency":T28, "TCP config":T29, "PRF (Hz)":dbl}
  T31 = enum16{"Init Program", "Init Hardware", "Main", "Reset", "Shutdown"}
  T32 = typedef "MicroPulse_Driver.lvlib/MP - scan data info.ctl" = cluster{"Message Header":u16, "Error Message":u16, "Test No.":u32, "Channel No.":u8, "Sweep No.":u32, "Gate No.":u32, "DOF":T33, "retain data":T34, "scan data":u16[], "scan length":i32, "scan index":i32, "peak data":cluster{"timebase":u16[], "data":u16[]}, "#peaks":i32, "PRF":dbl, "IP":cluster{"Axis No.":u8, "Location":u32, "MIP location":u32, "MIP?":bool}, "echo range":u16, "ETG":bool, "CAL 0 complete":bool, "Axis Positions":T35}
  T33 = typedef "MicroPulse_Driver.lvlib/MP - data output format.ctl" = enum16{"", "8-bit Mode", "10-bit Mode", "12-bit Mode", "16-bit Mode", "8-bit Log Mode", "12-bit Packed Mode"}
  T34 = typedef "MicroPulse_Driver.lvlib/MP - retain scan.ctl" = enum16{"None", "Ascan", "Peaks"}
  T35 = typedef "MicroPulse_Driver.lvlib/MP - axis positions (LLC).ctl" = cluster{"Axis 1":u32, "Axis 2":u32, "Axis 3":u32, "Axis 4":u32, "Status":u8}
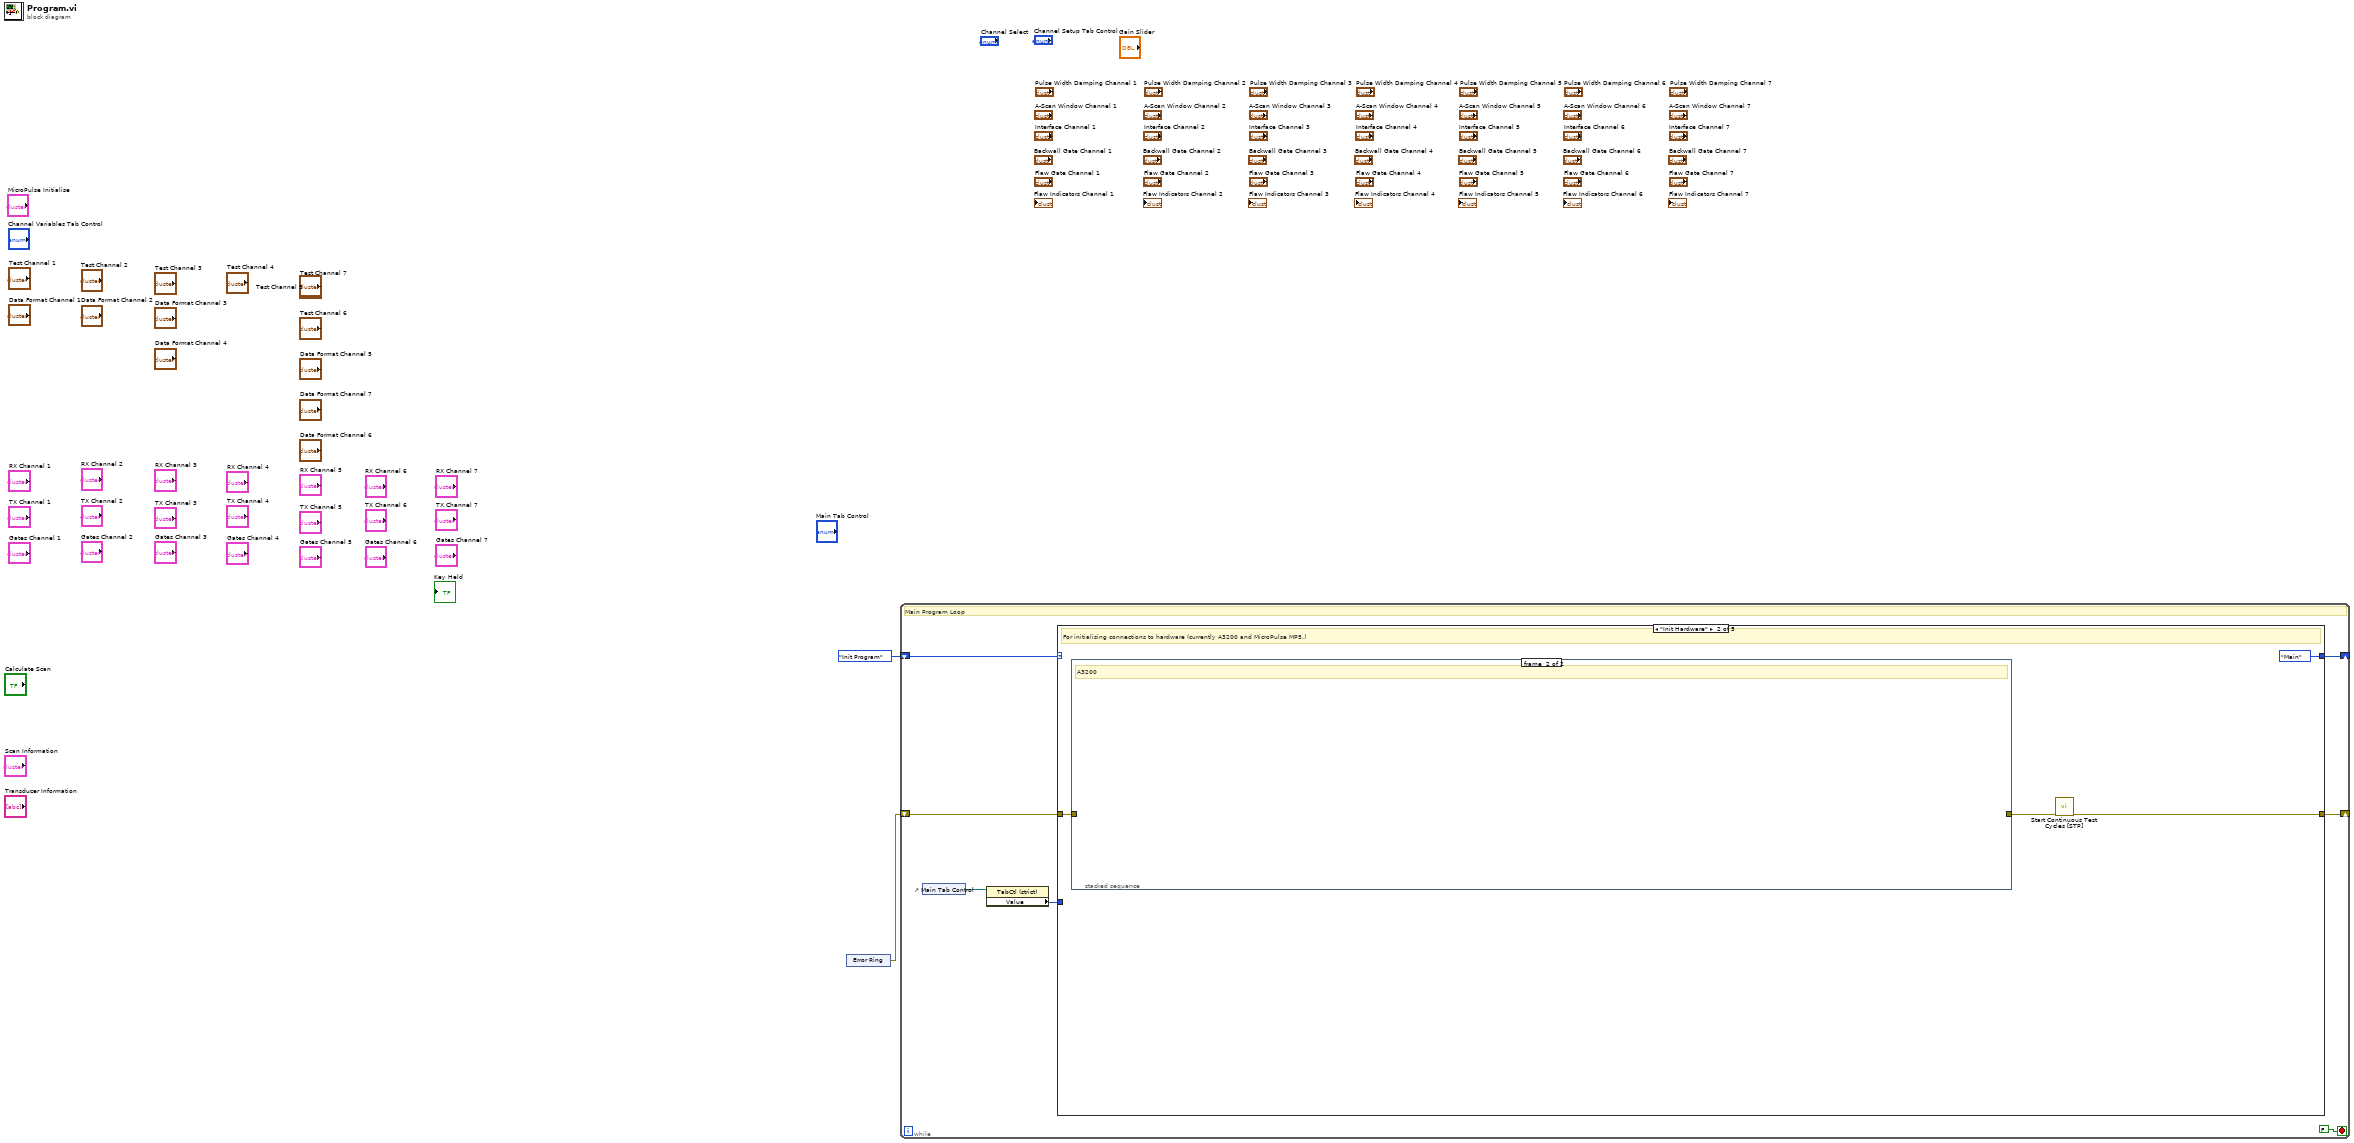
[diagram p0: block diagram]
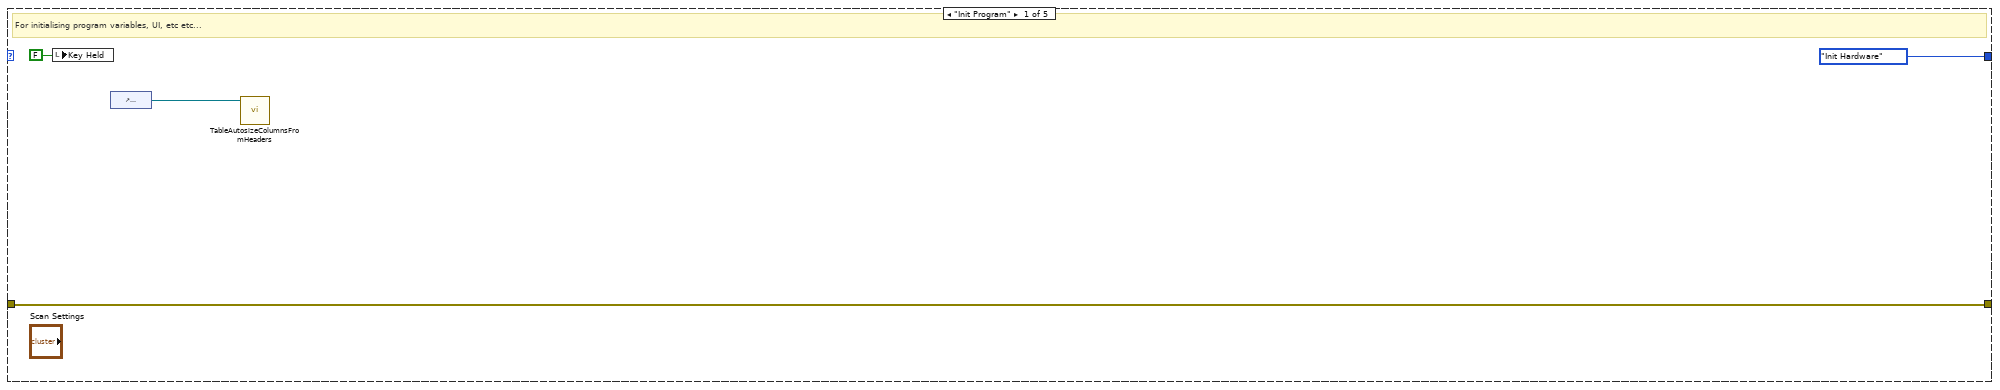
[diagram p2: hidden frame]
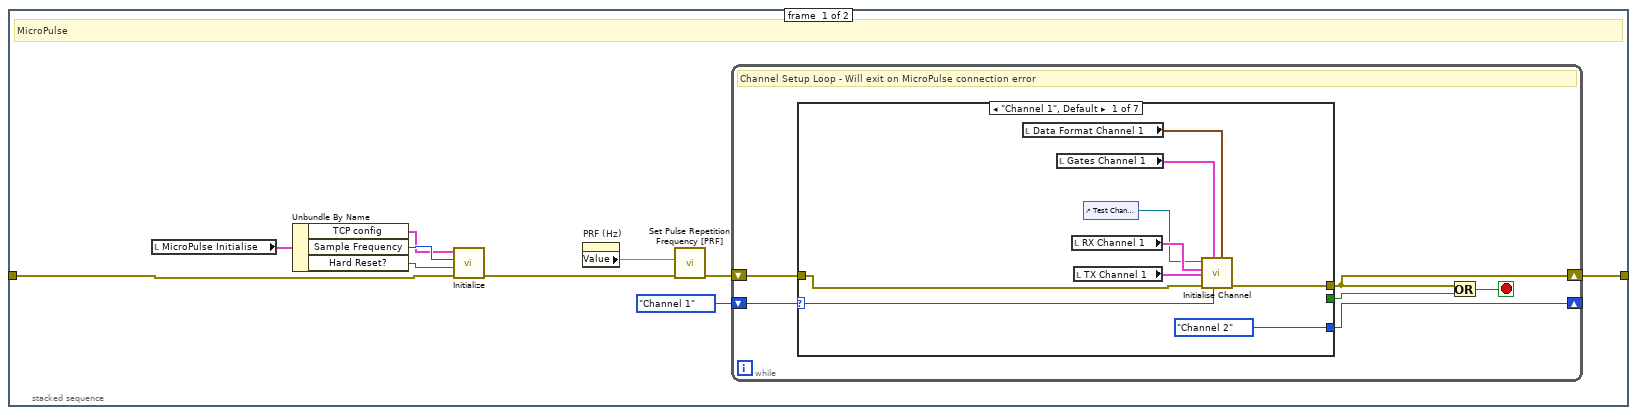
[diagram p3: hidden frame]
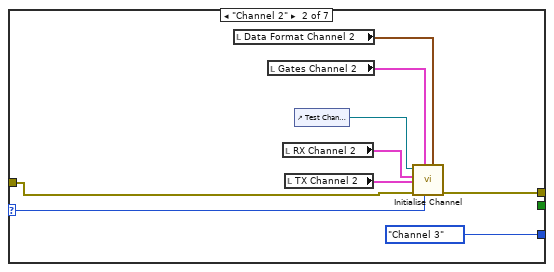
[diagram p4: hidden frame]
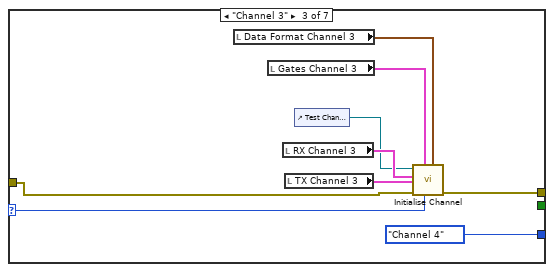
[diagram p5: hidden frame]
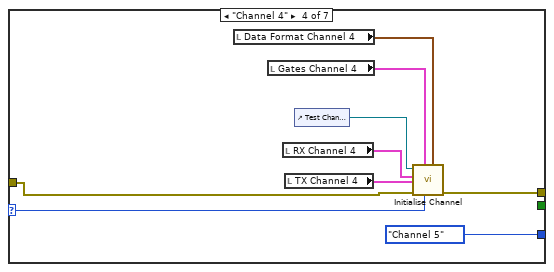
[diagram p6: hidden frame]
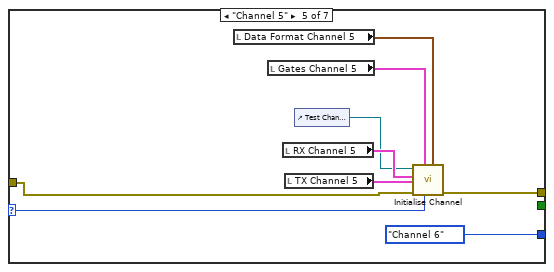
[diagram p7: hidden frame]
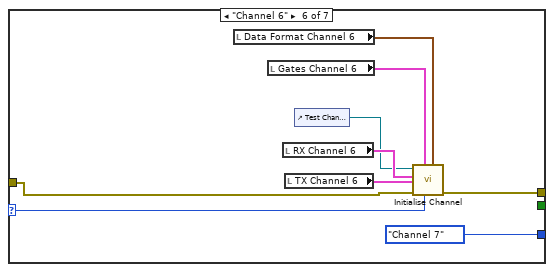
[diagram p8: hidden frame]
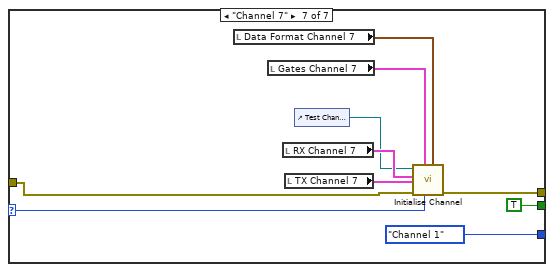
[diagram p9: hidden frame]
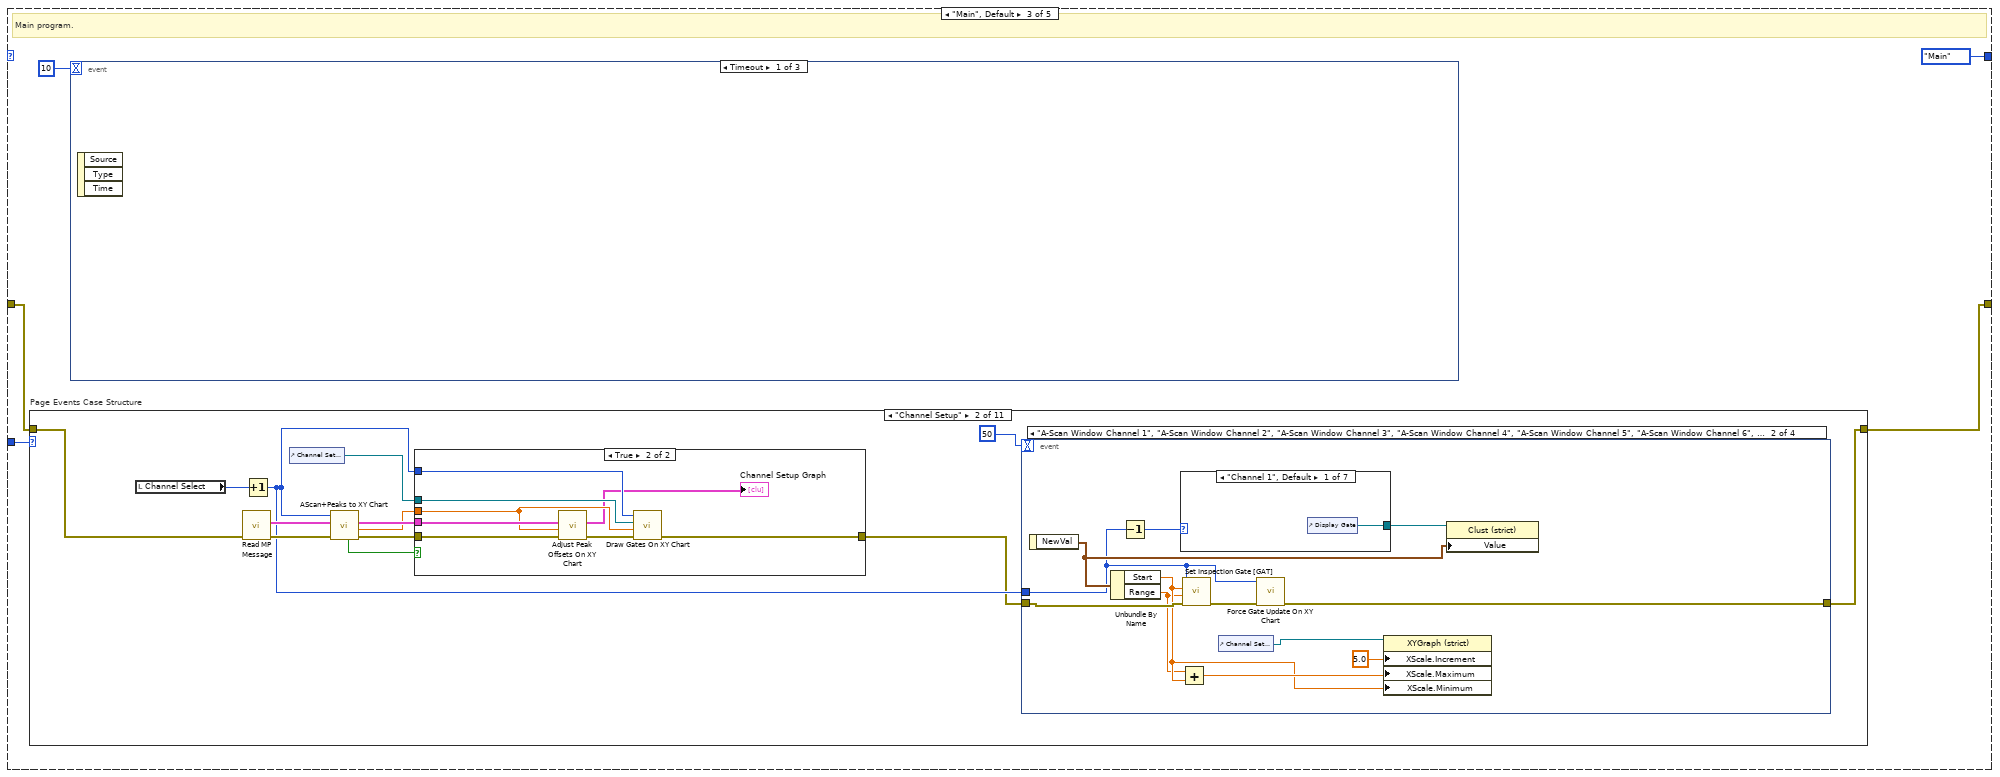
[diagram p10: hidden frame]
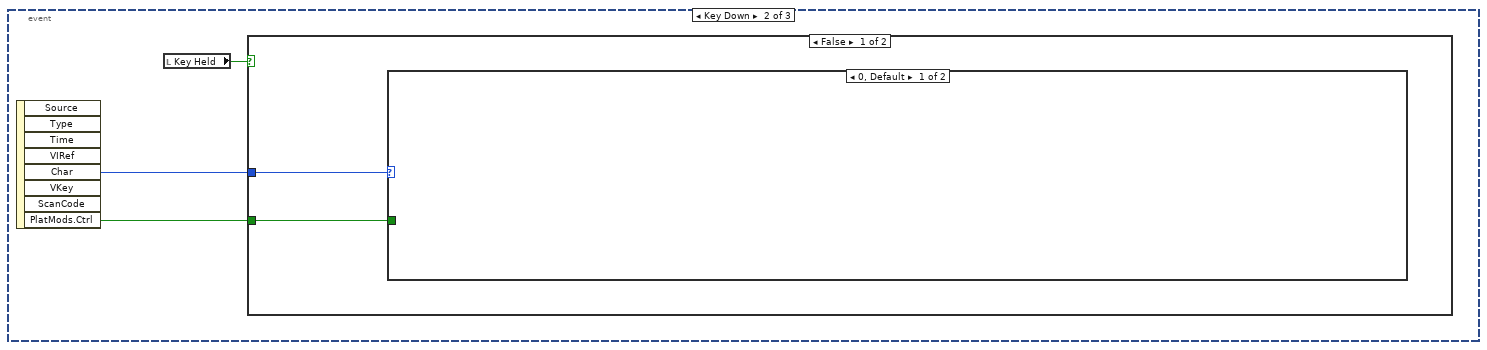
[diagram p11: hidden frame]
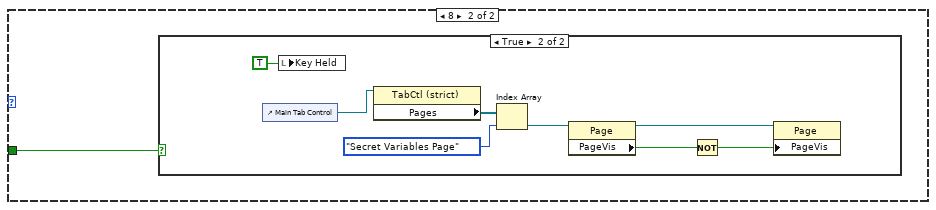
[diagram p12: hidden frame]
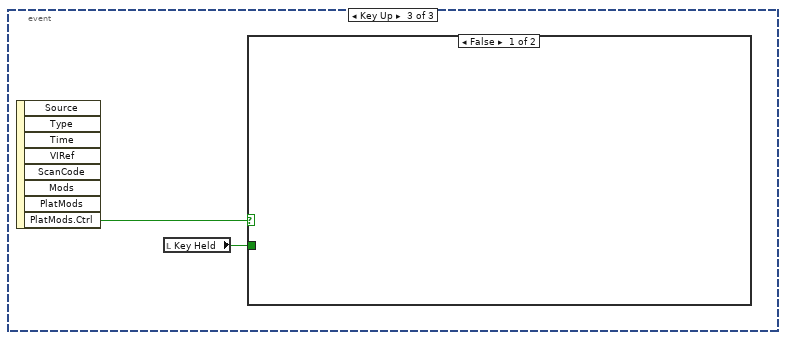
[diagram p15: hidden frame]
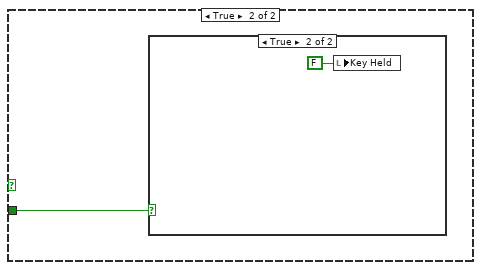
[diagram p16: hidden frame]
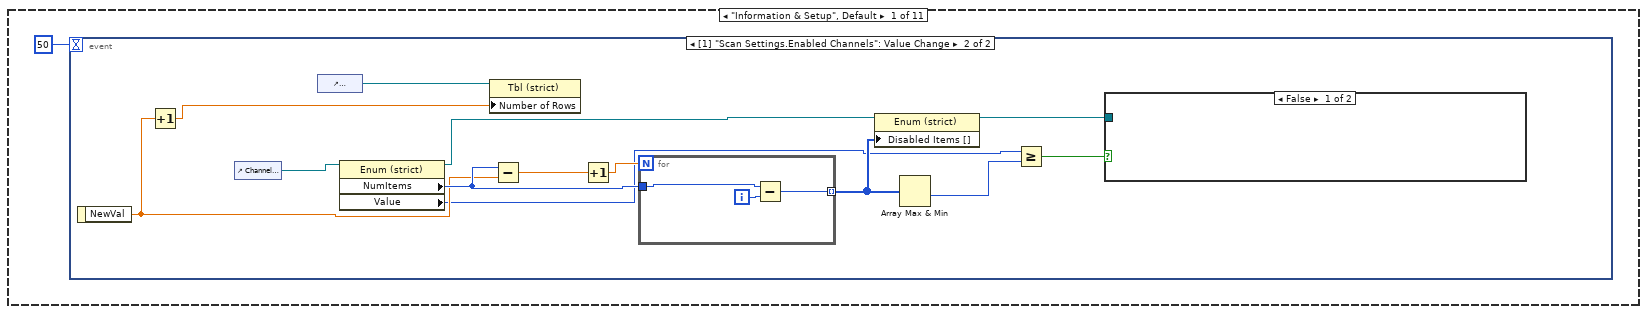
[diagram p18: hidden frame]
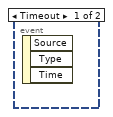
[diagram p19: hidden frame]
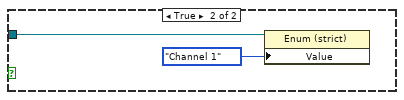
[diagram p20: hidden frame]
diagram:
  n1 = xnode "Error Ring"() -> ("error out"=w1:errorcluster)
  n2 = while {
    shift-right: [w8] -> _
    shift-left: T31."Init Program" -> [w9]
    shift-right: [w3] -> _
    shift-left: w1 -> [w4]
    stop <- FALSE stop-if-true
    # "Main Program Loop"
    n3 = control-ref of="Main Tab Control"() -> (w6:refnum<vi>)
    n4 = property class="TabCtl (strict)"(reference=w6) -> ("Value"=w5:T1)  [unwired: 1 in, 2 out]
    n5 = case shown="\"Init Hardware\"" w9 {
      tunnel: [T31."Init Hardware" T31."Main" T31."Main" _ _] -> w8
      tunnel: w5 -> [_ _ w102 _ _]
      tunnel: w4 -> [w10 w16 w99 w222 w223]
      tunnel: [w10 w14 w98 w222 w223] -> w3
      frame "Init Program" {
        # "For initialising program variables, UI, etc etc..."
        n6 = local write "Key Held"(FALSE ("Key Held")) -> ()
        n7 = control-ref of="Transducer Information"() -> (w13:refnum<vi>)
        n8 = call "TableAutosizeColumnsFromHeaders.vi"("Table in"=w13) -> ()  [unwired: 11 in]
      }
      frame "Init Hardware" {
        # "For initialising connections to hardware (currently A3200 and MicroPulse MP5.)"
        n9 = stacked-sequence {
          tunnel: w16 -> [w23 _]
          tunnel: [w21 _] -> w15
          frame #0 {
            # "MicroPulse"
            n10 = local read "MicroPulse Initialise"() -> (w27:T30)
            n11 = Unbundle By Name(w27) -> ("TCP config"=w24:T29, "Sample Frequency"=w25:T28, "Hard Reset?"=w26:bool)
            n12 = call <instrlib>:"Initialize.vi"("error in (no error)"=w23, "Hard Reset?"=w26, "Sample Frequency"=w25, "TCP config"=w24) -> ("error out"=w18:errorcluster)  [unwired: 6 in, 1 out]
            n13 = property on="PRF (Hz)" class="DigNum (strict)"() -> ("Value"=w20:dbl)  [unwired: 2 in, 2 out]
            n14 = call <instrlib>:"Set Pulse Repetition Frequency [PRF].vi"("error in (no error)"=w18, "Frequency (Hz)"=w20) -> ("error out"=w19:errorcluster)  [unwired: 8 in, 1 out]
            n15 = while {
              shift-right: [w29] -> w21
              shift-left: w19 -> [w33]
              shift-right: [w31] -> _
              shift-left: T10."Channel 1" ("Channel Select") -> [w32]
              stop <- w28 stop-if-true
              # "Channel Setup Loop - Will exit on MicroPulse connection error"
              n16 = case shown="\"Channel 1\", Default" w32 {
                selector: w32 -> [w34 w44 w57 w68 w76 w86 w94]
                tunnel: w33 -> [w41 w47 w56 w67 w77 w85 w95]
                tunnel: [w36 w43 w52 w61 w75 w84 w93] -> w29
                tunnel: [_ _ _ _ _ _ TRUE] -> w30
                tunnel: [T10."Channel 2" ("Channel Select") T10."Channel 3" ("Channel Select") T10."Channel 4" ("Channel Select") T10."Channel 5" ("Channel Select") T10."Channel 6" ("Channel Select") T10."Channel 7" ("Channel Select") T10."Channel 1" ("Channel Select")] -> w31
                frame "Channel 1", Default {
                  n17 = local read "Data Format Channel 1"() -> (w37:T21)
                  n18 = local read "Gates Channel 1"() -> (w38:T24)
                  n19 = local read "RX Channel 1"() -> (w40:T11)
                  n20 = local read "TX Channel 1"() -> (w39:T19)
                  n21 = control-ref of="Test Channel 1"() -> (w35:refnum<vi>)
                  n22 = call "Initialise Channel.vi"("Data Format In"=w37, "Channel In"=w34, "Gates In"=w38, "error in (no error)"=w41, "Transmit In (TX)"=w39, "Recieve In (RX)"=w40, "Test Reference In"=w35) -> ("error out"=w36:errorcluster)  [unwired: 4 in]
                }
                frame "Channel 2" {
                  n23 = local read "Data Format Channel 2"() -> (w45:T21)
                  n24 = local read "Gates Channel 2"() -> (w46:T24)
                  n25 = local read "RX Channel 2"() -> (w48:T11)
                  n26 = local read "TX Channel 2"() -> (w49:T19)
                  n27 = control-ref of="Test Channel 2"() -> (w50:refnum<vi>)
                  n28 = call "Initialise Channel.vi"("Data Format In"=w45, "Channel In"=w44, "Gates In"=w46, "error in (no error)"=w47, "Transmit In (TX)"=w49, "Recieve In (RX)"=w48, "Test Reference In"=w50) -> ("error out"=w43:errorcluster)  [unwired: 4 in]
                }
                frame "Channel 3" {
                  n29 = local read "Data Format Channel 3"() -> (w58:T21)
                  n30 = local read "Gates Channel 3"() -> (w59:T24)
                  n31 = local read "RX Channel 3"() -> (w54:T11)
                  n32 = local read "TX Channel 3"() -> (w55:T19)
                  n33 = control-ref of="Test Channel 3"() -> (w53:refnum<vi>)
                  n34 = call "Initialise Channel.vi"("Data Format In"=w58, "Channel In"=w57, "Gates In"=w59, "error in (no error)"=w56, "Transmit In (TX)"=w55, "Recieve In (RX)"=w54, "Test Reference In"=w53) -> ("error out"=w52:errorcluster)  [unwired: 4 in]
                }
                frame "Channel 4" {
                  n35 = local read "Data Format Channel 4"() -> (w62:T21)
                  n36 = local read "Gates Channel 4"() -> (w63:T24)
                  n37 = local read "RX Channel 4"() -> (w65:T11)
                  n38 = local read "TX Channel 4"() -> (w64:T19)
                  n39 = control-ref of="Test Channel 4"() -> (w66:refnum<vi>)
                  n40 = call "Initialise Channel.vi"("Data Format In"=w62, "Channel In"=w68, "Gates In"=w63, "error in (no error)"=w67, "Transmit In (TX)"=w64, "Recieve In (RX)"=w65, "Test Reference In"=w66) -> ("error out"=w61:errorcluster)  [unwired: 4 in]
                }
                frame "Channel 5" {
                  n41 = local read "Data Format Channel 5"() -> (w72:T21)
                  n42 = local read "Gates Channel 5"() -> (w73:T24)
                  n43 = local read "RX Channel 5"() -> (w74:T11)
                  n44 = local read "TX Channel 5"() -> (w71:T19)
                  n45 = control-ref of="Test Channel 5"() -> (w70:refnum<vi>)
                  n46 = call "Initialise Channel.vi"("Data Format In"=w72, "Channel In"=w76, "Gates In"=w73, "error in (no error)"=w77, "Transmit In (TX)"=w71, "Recieve In (RX)"=w74, "Test Reference In"=w70) -> ("error out"=w75:errorcluster)  [unwired: 4 in]
                }
                frame "Channel 6" {
                  n47 = local read "Data Format Channel 6"() -> (w83:T21)
                  n48 = local read "Gates Channel 6"() -> (w82:T24)
                  n49 = local read "RX Channel 6"() -> (w81:T11)
                  n50 = local read "TX Channel 6"() -> (w80:T19)
                  n51 = control-ref of="Test Channel 6"() -> (w79:refnum<vi>)
                  n52 = call "Initialise Channel.vi"("Data Format In"=w83, "Channel In"=w86, "Gates In"=w82, "error in (no error)"=w85, "Transmit In (TX)"=w80, "Recieve In (RX)"=w81, "Test Reference In"=w79) -> ("error out"=w84:errorcluster)  [unwired: 4 in]
                }
                frame "Channel 7" {
                  n53 = local read "Data Format Channel 7"() -> (w92:T21)
                  n54 = local read "Gates Channel 7"() -> (w91:T24)
                  n55 = local read "RX Channel 7"() -> (w90:T11)
                  n56 = local read "TX Channel 7"() -> (w89:T19)
                  n57 = control-ref of="Test Channel 7"() -> (w88:refnum<vi>)
                  n58 = call "Initialise Channel.vi"("Data Format In"=w92, "Channel In"=w94, "Gates In"=w91, "error in (no error)"=w95, "Transmit In (TX)"=w89, "Recieve In (RX)"=w90, "Test Reference In"=w88) -> ("error out"=w93:errorcluster)  [unwired: 4 in]
                }
              }
              n59 = Or(x=w29, y=w30) -> (x .or. y?=w28:bool)
            }
          }
          frame #1 {
            # "A3200"
          }
        }
        n60 = call <instrlib>:"Start Continuous Test Cycles [STP].vi"("error in (no error)"=w15) -> ("error out"=w14:errorcluster)  [unwired: 9 in, 1 out]
      }
      frame "Main", Default {
        # "Main program."
        n61 = case "Page Events Case Structure" shown="\"Channel Setup\"" w102 {
          tunnel: w99 -> [_ w142 w221 _ _ _ _ _ _ _ _]
          tunnel: [_ w140 w221 _ _ _ _ _ _ _ _] -> w98
          frame "Information & Setup", Default {
            n62 = event shown="[1] \"Scan Settings.Enabled Channels\": Value Change" {
              selector: _ -> [_ _]
              dyn-events: _ -> [_ _]
              timeout: 50 -> [_ _]
              event Timeout {
                n63 = event-data() -> ()  [unwired: 1 in, 3 out]
              }
              event "Scan Settings.Enabled Channels": Value Change {
                n64 = event-data() -> ("NewVal"=w128:dbl)  [unwired: 1 in]
                n65 = Increment(x=w128) -> (x+1=w129:dbl)
                n66 = control-ref of="Channel Select"() -> (w131:refnum<vi>)
                n67 = control-ref of="Transducer Information"() -> (w130:refnum<vi>)
                n68 = property class="Enum (strict)"(reference=w131) -> (reference out=w134:refnum<vi>, "NumItems"=w133:u32, "Value"=w125:T10)  [unwired: 1 in, 1 out]
                n69 = property class="Tbl (strict)"(reference=w130, "Number of Rows"=w129) -> ()  [unwired: 1 in, 2 out]
                n70 = Subtract(x=w133, y=w128) -> (x-y=w132:dbl)
                n71 = Increment(x=w132) -> (x+1=w127:dbl)
                n72 = for {
                  N: w127 -> [_]
                  tunnel: w133 -> [w139]
                  tunnel: [w137] -> w126 mode=indexing
                  i -> [w138]
                  n73 = Subtract(x=w139, y=w138) -> (x-y=w137:u32)
                }
                n74 = property class="Enum (strict)"(reference=w134, "Disabled Items []"=w126) -> (reference out=w122:refnum<vi>)  [unwired: 1 in, 1 out]
                n75 = Array Max & Min(array=w126) -> (min value=w124:u32)  [unwired: 3 out]
                n76 = Greater Or Equal?(x=w125, y=w124) -> (x >= y?=w123:bool)
                n77 = case shown="False" w123 {
                  tunnel: w122 -> [_ w136]
                  frame False {
                  }
                  frame True {
                    n78 = property class="Enum (strict)"(reference=w136, "Value"=T10."Channel 1") -> ()  [unwired: 1 in, 2 out]
                  }
                }
              }
            }
          }
          frame "Channel Setup" {
            n79 = local read "Channel Select"() -> (w149:T10)
            n80 = call <instrlib>:"Read MP Message.vi"("error in (no error)"=w142) -> ("error out"=w150:errorcluster, "scan data info"=w151:T32)  [unwired: 6 in, 3 out]
            n81 = Increment(x=w149) -> (x+1=w143:T10)
            n82 = control-ref of="Channel Setup Graph"() -> (w144:refnum<vi>)
            n83 = call <instrlib>:"AScan+Peaks to XY Chart.vi"("error in (no error)"=w150, "scan data info"=w151, "Test No."=w143) -> ("error out"=w147:errorcluster, "Echo Range (us)"=w145:dbl, "AScan+Peaks"=w146:cluster{"timebase":dbl[], "data":u16[]}[], "Update Indicators?"=w148:bool)  [unwired: 3 in, 2 out]
            n84 = case shown="True" w148 {
              tunnel: w147 -> [w153 w161]
              tunnel: [w153 w159] -> w141
              tunnel: w143 -> [_ w158]
              tunnel: w146 -> [_ w157]
              tunnel: w145 -> [_ w156]
              tunnel: w144 -> [_ w155]
              frame False {
              }
              frame True {
                n85 = call <instrlib>:"Adjust Peak Offsets On XY Chart.vi"("error in (no error)"=w161, "Echo Range in"=w156, "AScan+Peaks in"=w157) -> ("error out"=w160:errorcluster, "AScan+Peaks out"=→"Channel Setup Graph":cluster{"timebase":dbl[], "data":u16[]}[])  [unwired: 7 in]
                n86 = call <instrlib>:"Draw Gates On XY Chart.vi"("error in (no error)"=w160, "Echo Range"=w156, "XYGraph in"=w155, "Test No."=w158) -> ("error out"=w159:errorcluster)  [unwired: 7 in]
              }
            }
            n87 = event shown="[1] \"A-Scan Window Channel 1\", \"A-Scan Window Channel 2\", \"A-Scan Window Channel 3\", \"A-Scan Window Channel 4\", \"A-Scan Window Channel 5\", \"A-Scan Window Channel 6\", \"A-Scan Window Channel 7\": Value Change" {
              selector: _ -> [_ _ _ _]
              dyn-events: _ -> [_ _ _ _]
              timeout: 50 -> [_ _ _ _]
              tunnel: w143 -> [_ w162 w183 w210]
              tunnel: w141 -> [_ w171 w182 w208]
              tunnel: [_ w163 w181 w207] -> w140
              event Timeout {
                n88 = event-data() -> ()  [unwired: 1 in, 3 out]
              }
              event "A-Scan Window Channel 1", "A-Scan Window Channel 2", "A-Scan Window Channel 3", "A-Scan Window Channel 4", "A-Scan Window Channel 5", "A-Scan Window Channel 6", "A-Scan Window Channel 7": Value Change {
                n89 = event-data() -> ("NewVal"=w172:cluster{"Start":dbl, "Range":dbl})  [unwired: 1 in]
                n90 = Unbundle By Name(w172) -> ("Start"=w165:dbl, "Range"=w164:dbl)
                n91 = Decrement(x=w162) -> (x-1=w169:T10)
                n92 = Add(x=w164, y=w165) -> (x+y=w166:dbl)
                n93 = case shown="\"Channel 1\", Default" w169 {
                  tunnel: [w174 w175 w176 w177 w178 w179 w180] -> w173
                  frame "Channel 1", Default {
                    n94 = control-ref of="Display Gate"() -> (w174:refnum<vi>)
                  }
                  frame "Channel 2" {
                    n95 = control-ref of="Display Gate"() -> (w175:refnum<vi>)
                  }
                  frame "Channel 3" {
                    n96 = control-ref of="Display Gate"() -> (w176:refnum<vi>)
                  }
                  frame "Channel 4" {
                    n97 = control-ref of="Display Gate"() -> (w177:refnum<vi>)
                  }
                  frame "Channel 5" {
                    n98 = control-ref of="Display Gate"() -> (w178:refnum<vi>)
                  }
                  frame "Channel 6" {
                    n99 = control-ref of="Display Gate"() -> (w179:refnum<vi>)
                  }
                  frame "Channel 7" {
                    n100 = control-ref of="Display Gate"() -> (w180:refnum<vi>)
                  }
                }
                n101 = call <instrlib>:"Set Inspection Gate [GAT].vi"("error in (no error)"=w171, "Gate Length (us)"=w164, "Gate Start (us)"=w165, "Test Number"=w162) -> ("error out"=w170:errorcluster)  [unwired: 6 in, 1 out]
                n102 = control-ref of="Channel Setup Graph"() -> (w168:refnum<vi>)
                n103 = call <instrlib>:"Force Gate Update On XY Chart.vi"("error in (no error)"=w170, "Test No."=w162) -> ("error out"=w163:errorcluster)  [unwired: 7 in, 2 out]
                n104 = property class="XYGraph (strict)"(reference=w168, "XScale.Increment"=5.0 ("X Scale.Range:Increment"), "XScale.Maximum"=w166, "XScale.Minimum"=w165) -> ()  [unwired: 1 in, 2 out]
                n105 = property class="Clust (strict)"(reference=w173, "Value"=w172) -> ()  [unwired: 1 in, 2 out]
              }
              event "Channel Select": Value Change {
                n106 = event-data() -> ("NewVal"=w191:T10)  [unwired: 1 in]
                n107 = case shown="\"Channel 7\"" w191 {
                  tunnel: [w194 w196 w198 w200 w202 w204 w206] -> w190
                  tunnel: [w193 w195 w197 w199 w201 w203 w205] -> w184
                  frame "Channel 1", Default {
                    n108 = local read "A-Scan Window Channel 1"() -> (w194:cluster{"Start":dbl, "Range":dbl})
                    n109 = property on="Gain" class="DigNum (strict)"() -> ("Value"=w193:dbl)  [unwired: 2 in, 2 out]
                  }
                  frame "Channel 2" {
                    n110 = local read "A-Scan Window Channel 2"() -> (w196:cluster{"Start":dbl, "Range":dbl})
                    n111 = property on="Gain" class="DigNum (strict)"() -> ("Value"=w195:dbl)  [unwired: 2 in, 2 out]
                  }
                  frame "Channel 3" {
                    n112 = local read "A-Scan Window Channel 3"() -> (w198:cluster{"Start":dbl, "Range":dbl})
                    n113 = property on="Gain" class="DigNum (strict)"() -> ("Value"=w197:dbl)  [unwired: 2 in, 2 out]
                  }
                  frame "Channel 4" {
                    n114 = local read "A-Scan Window Channel 4"() -> (w200:cluster{"Start":dbl, "Range":dbl})
                    n115 = property on="Gain" class="DigNum (strict)"() -> ("Value"=w199:dbl)  [unwired: 2 in, 2 out]
                  }
                  frame "Channel 5" {
                    n116 = local read "A-Scan Window Channel 5"() -> (w202:cluster{"Start":dbl, "Range":dbl})
                    n117 = property on="Gain" class="DigNum (strict)"() -> ("Value"=w201:dbl)  [unwired: 2 in, 2 out]
                  }
                  frame "Channel 6" {
                    n118 = local read "A-Scan Window Channel 6"() -> (w204:cluster{"Start":dbl, "Range":dbl})
                    n119 = property on="Gain" class="DigNum (strict)"() -> ("Value"=w203:dbl)  [unwired: 2 in, 2 out]
                  }
                  frame "Channel 7" {
                    n120 = local read "A-Scan Window Channel 7"() -> (w206:cluster{"Start":dbl, "Range":dbl})
                    n121 = property on="Gain" class="DigNum (strict)"() -> ("Value"=w205:dbl)  [unwired: 2 in, 2 out]
                  }
                }
                n122 = call <instrlib>:"Force Gate Update On XY Chart.vi"("error in (no error)"=w182, "Test No."=w183) -> ("error out"=w181:errorcluster)  [unwired: 7 in, 2 out]
                n123 = control-ref of="Channel Setup Tab Control"() -> (w192:refnum<vi>)
                n124 = property class="TabCtl (strict)"(reference=w192, "Value"=w191) -> ()  [unwired: 1 in, 2 out]
                n125 = control-ref of="Channel Setup Graph"() -> (w185:refnum<vi>)
                n126 = local write "Gain Slider"(w184) -> ()
                n127 = Unbundle By Name(w190) -> ("Start"=w189:dbl, "Range"=w188:dbl)
                n128 = Add(x=w189, y=w188) -> (x+y=w187:dbl)
                n129 = property class="XYGraph (strict)"(reference=w185, "XScale.Increment"=5.0 ("X Scale.Range:Increment"), "XScale.Minimum"=w189, "XScale.Maximum"=w187) -> ()  [unwired: 1 in, 2 out]
              }
              event "Gain Slider": Value Change {
                n130 = event-data() -> ("NewVal"=w209:dbl)  [unwired: 1 in, 5 out]
                n131 = call <instrlib>:"Set Gain [GAN].vi"("error in (no error)"=w208, "Gain (dB)"=w209, "Test Number"=w210) -> ("error out"=w207:errorcluster)  [unwired: 7 in, 1 out]
                n132 = control-ref of="Channel Select"() -> (w213:refnum<vi>)
                n133 = property class="Enum (strict)"(reference=w213) -> ("Value"=w212:T10)  [unwired: 1 in, 2 out]
                n134 = case shown="\"Channel 2\"" w212 {
                  tunnel: [w214 w215 w216 w217 w218 w219 w220] -> w211
                  frame "Channel 1", Default {
                    n135 = control-ref of="Gain"() -> (w214:refnum<vi>)
                  }
                  frame "Channel 2" {
                    n136 = control-ref of="Gain"() -> (w215:refnum<vi>)
                  }
                  frame "Channel 3" {
                    n137 = control-ref of="Gain"() -> (w216:refnum<vi>)
                  }
                  frame "Channel 4" {
                    n138 = control-ref of="Gain"() -> (w217:refnum<vi>)
                  }
                  frame "Channel 5" {
                    n139 = control-ref of="Gain"() -> (w218:refnum<vi>)
                  }
                  frame "Channel 6" {
                    n140 = control-ref of="Gain"() -> (w219:refnum<vi>)
                  }
                  frame "Channel 7" {
                    n141 = control-ref of="Gain"() -> (w220:refnum<vi>)
                  }
                }
                n142 = property class="DigNum (strict)"(reference=w211, "Value"=w209) -> ()  [unwired: 1 in, 2 out]
              }
            }
          }
          frame "Beam Width" {
          }
          frame "C-Scan" {
          }
          frame "Analysis Results" {
          }
          frame "Auto SNR Analysis" {
          }
          frame "Heat Details" {
          }
          frame "Reporting Page" {
          }
          frame "System Diagnostics" {
          }
          frame "Alignment Check" {
          }
          frame "Secret Variables Page" {
          }
        }
        n143 = event shown="[0] Timeout" {
          selector: _ -> [_ _ _]
          dyn-events: _ -> [_ _ _]
          timeout: 10 -> [_ _ _]
          event Timeout {
            n144 = event-data() -> ()  [unwired: 1 in, 3 out]
          }
          event Key Down {
            n145 = event-data() -> ("Char"=w105:i16, "PlatMods.Ctrl"=w104:bool)  [unwired: 1 in, 6 out]
            n146 = local read "Key Held"() -> (w103:bool)
            n147 = case shown="False" w103 {
              tunnel: w105 -> [w107 _]
              tunnel: w104 -> [w106 _]
              frame False {
                n148 = case shown="0, Default" w107 {
                  tunnel: w106 -> [_ w108]
                  frame 0, Default {
                  }
                  frame 8 {
                    n149 = case shown="True" w108 {
                      frame False {
                      }
                      frame True {
                        n150 = control-ref of="Main Tab Control"() -> (w111:refnum<vi>)
                        n151 = local write "Key Held"(TRUE ("Key Held")) -> ()
                        n152 = property class="TabCtl (strict)"(reference=w111) -> ("Pages"=w112:refnum<vi>[])  [unwired: 1 in, 2 out]
                        n153 = Index Array(array=w112, index=T1."Secret Variables Page" ("Value")) -> (element=w113:refnum<vi>)
                        n154 = property class="Page"(reference=w113) -> (reference out=w116:refnum<vi>, "PageVis"=w115:bool)  [unwired: 1 in, 1 out]
                        n155 = Not(x=w115) -> (.not. x?=w114:bool)
                        n156 = property class="Page"(reference=w116, "PageVis"=w114) -> ()  [unwired: 1 in, 2 out]
                      }
                    }
                  }
                }
              }
              frame True {
              }
            }
          }
          event Key Up {
            n157 = event-data() -> ("PlatMods.Ctrl"=w117:bool)  [unwired: 1 in, 7 out]
            n158 = local read "Key Held"() -> (w118:bool)
            n159 = case shown="False" w117 {
              tunnel: w118 -> [_ w119]
              frame False {
              }
              frame True {
                n160 = case shown="True" w119 {
                  frame False {
                  }
                  frame True {
                    n161 = local write "Key Held"(FALSE ("Key Held")) -> ()
                  }
                }
              }
            }
          }
        }
      }
      frame "Reset" {
      }
      frame "Shutdown" {
      }
    }
  }
